vi "Display n or dt.vi"(8 "error in (no error)":errorcluster, 9 "Display n?":bool, 11 "Input Waveforms":waveform(dbl)[](array[waveform])) -> (0 "error out":errorcluster, 3 "Output Waveforms":waveform(dbl)[](array[waveform]))   [LabVIEW 2016, in "Instrument.Lockin.lvclass"]
uses:
  Instrument.Lockin.lvclass
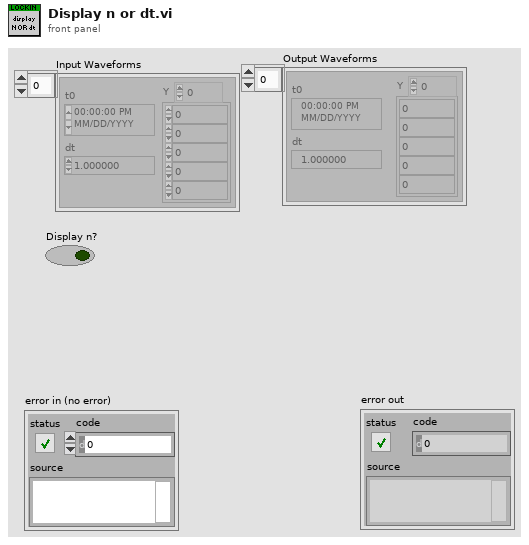
[diagram p1: front panel]
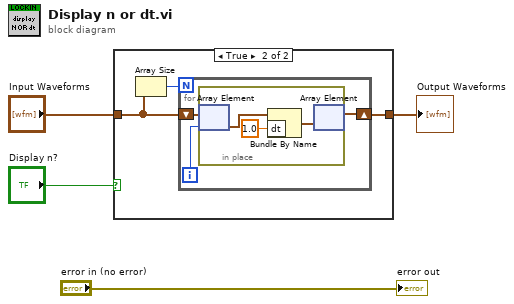
[diagram p0: block diagram]
diagram:
  n1 = case shown="True" "Display n?" {
    tunnel: [w5 w8] -> w4
    tunnel: "Input Waveforms" -> [w5 w6]
    frame False {
    }
    frame True {
      n2 = Array Size(array=w6) -> (size(s)=w7:i32)
      n3 = for {
        N: w7 -> [_]
        shift-right: [w9] -> w8
        shift-left: w6 -> [w10]
        i -> [w11]
        n4 = in-place {
          n5 = in-place-array #1(w10, w11) -> (w12:waveform(dbl))
          n6 = Bundle By Name(cluster=w12, "dt"=1.0) -> (w13:waveform(dbl))
          n7 = in-place-array #1(w13) -> (w9:waveform(dbl)[])  [unwired: 1 out]
        }
      }
    }
  }
  "Output Waveforms" <- w4
  "error out" <- "error in (no error)"
